vi "Test Gradient Ascent.vi"() -> ()   [LabVIEW 2014]
panel:
  in  "Focus Parameters":T1
  out "XY Graph":cluster{"array":dbl[], "array":dbl[]}[](graph)
  in  "StepSize":dbl format="%#_13g"
  in  "Range Z":dbl format="%#_13g"
  in  "Alpha":dbl
  in  "Delta Z0":dbl format="%#_13g"
  # "LICENSED MATERIALS – PROPERTY OF IBM\nCopyright IBM Corp. 2016,\nALL RIGHTS RESERVED"
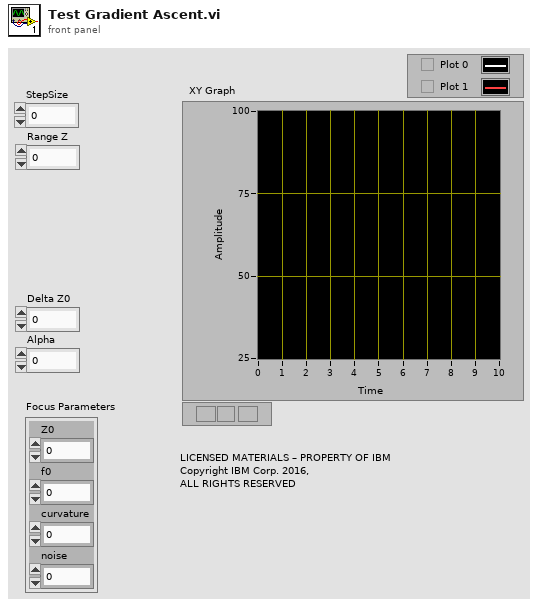
[diagram p1: front panel]
types:
  T1 = cluster{"Z0":dbl, "f0":dbl, "curvature":dbl, "noise":dbl}
  T2 = cluster{"Match":cluster{"Position":cluster{"x":sgl, "y":sgl}, "Angle":sgl, "Scale":sgl, "Score":sgl, "Bounding Box":cluster{"x":sgl, "y":sgl}[]}, "Edge Analysis":cluster{"Mean Value":sgl, "Standard Variation":sgl, "Minimal Value":sgl, "Maximal Value":sgl, "Area (calibrated)":sgl, "Area (pixels)":i32, "%":sgl}}
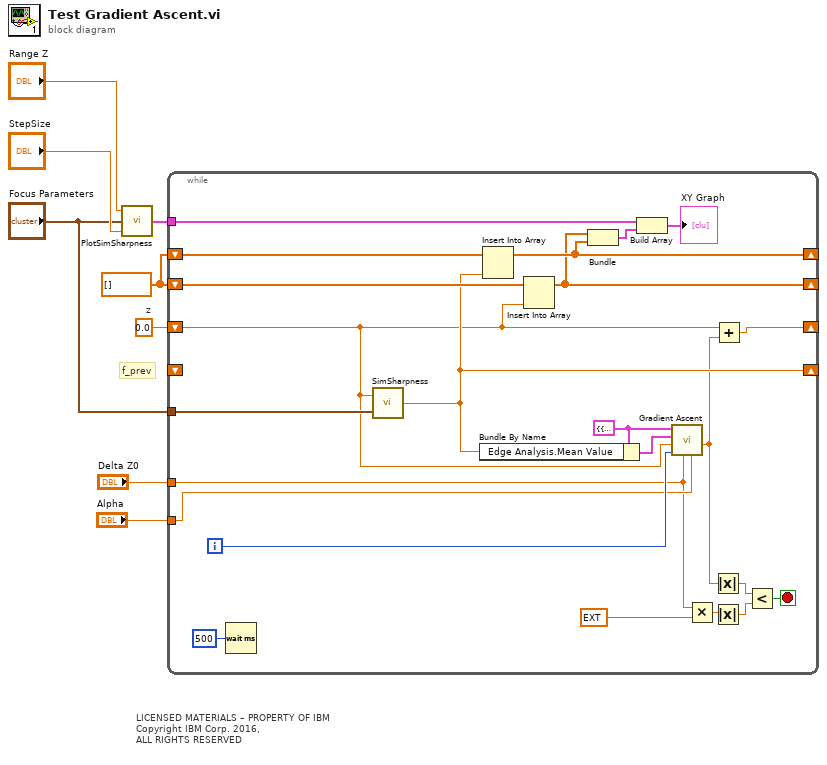
[diagram p0: block diagram]
diagram:
  w4 = dbl[] [] ("array")
  w5 = 0.0  # z
  # "LICENSED MATERIALS – PROPERTY OF IBM\nCopyright IBM Corp. 2016,\nALL RIGHTS RESERVED"
  # "f_prev"
  n1 = call "PlotSimSharpness.vi"("StepSize"="StepSize", "Focus Parameters"="Focus Parameters", "Range Z"="Range Z") -> ("Cluster"=w6:cluster{dbl[], dbl[]})
  n2 = while {
    tunnel: w6 -> [w31]
    shift-right: [w22] -> _
    shift-left: w5 -> [w9]
    tunnel: "Focus Parameters" -> [w23]
    shift-right: [w24] -> _
    shift-left: w4 -> [w29]
    shift-right: [w25] -> _
    shift-left: w4 -> [w27]
    shift-right: [w19] -> _
    shift-left: _ -> [_]
    tunnel: "Alpha" -> [w17]
    tunnel: "Delta Z0" -> [w16]
    i -> [w18]
    stop <- w10 stop-if-true
    w21 = T2 {"Match"={"Position"={"x"=0.0, "y"=0.0}, "Angle"=0.0, "Scale"=0.0, "Score"=0.0, "Bounding Box"=[]}, "Edge Analysis"={"Mean Value"=0.0, "Standard Variation"=0.0, "Minimal Value"=0.0, "Maximal Value"=0.0, "Area (calibrated)"=0.0, "Area (pixels)"=0, "%"=0.0}} ("Target Data")
    n3 = Wait (ms)(milliseconds to wait=u32 500) -> ()  [unwired: 1 out]
    n4 = call "SimSharpness.vi"("Focus Parameters"=w23, "Z"=w9) -> ("Sharpness"=w19:dbl)
    n5 = Bundle By Name(cluster=w21, "Edge Analysis.Mean Value"=w19) -> (w20:T2)
    n6 = Insert Into Array(array=w27, new element=w19) -> (w25:dbl[])  [unwired: 1 in]
    n7 = Insert Into Array(array=w29, new element=w9) -> (w24:dbl[])  [unwired: 1 in]
    n8 = Bundle("array"=w24, "array"=w25) -> (w28:cluster{"array":dbl[], "array":dbl[]})  [unwired: 1 in]
    n9 = Build Array(w31, w28) -> (→"XY Graph":cluster{"array":dbl[], "array":dbl[]}[])
    n10 = call "Gradient Ascent.vi"("Alpha"=w17, "Delta Z0"=w16, "Optimization Step"=w18, "Z"=w9, "Current Data"=w20, "Target Data"=w21) -> ("Delta Z"=w13:dbl)  [unwired: 4 in, 1 out]
    n11 = Multiply(x=w16, y=ext 0.01) -> (x*y=w14:ext)
    n12 = Absolute Value(x=w13) -> (abs(x)=w12:dbl)
    n13 = Absolute Value(x=w14) -> (abs(x)=w11:ext)
    n14 = Add(x=w9, y=w13) -> (x+y=w22:dbl)
    n15 = Less?(x=w12, y=w11) -> (x < y?=w10:bool)
  }
